vi "加载流程文件.vi"(8 "错误输入（无错误）":errorcluster) -> (0 "错误输出":errorcluster, 3 "流程":T1 {"进样流程"."进样流程-进样"."步骤二："."功能" items=["加标", "进样", "排液", "搅拌", "定量", "延时"]; "进样流程"."进样流程-进样"."步骤一："."功能" items=["加标", "进样", "排液", "搅拌", "定量", "延时"]; "进样流程"."进样流程-进样"."步骤四："."功能" items=["加标", "进样", "排液", "搅拌", "定量", "延时"]; "进样流程"."进样流程-进样"."步骤三："."功能" items=["加标", "进样", "排液", "搅拌", "定量", "延时"]; "进样流程"."进样流程-进样"."步骤六："."功能" items=["加标", "进样", "排液", "搅拌", "定量", "延时"]; "进样流程"."进样流程-进样"."步骤五："."功能" items=["加标", "进样", "排液", "搅拌", "定量", "延时"]; "进样流程"."进样流程-进样"."步骤八："."功能" items=["加标", "进样", "排液", "搅拌", "定量", "延时"]; "进样流程"."进样流程-进样"."步骤七："."功能" items=["加标", "进样", "排液", "搅拌", "定量", "延时"]; "进样流程"."进样流程-进样"."步骤十："."功能" items=["加标", "进样", "排液", "搅拌", "定量", "延时"]; "进样流程"."进样流程-进样"."步骤九："."功能" items=["加标", "进样", "排液", "搅拌", "定量", "延时"]; "进样流程"."进样流程-润洗"."步骤二："."功能" items=["加标", "进样", "排液", "搅拌", "定量", "延时"]; "进样流程"."进样流程-润洗"."步骤一："."功能" items=["加标", "进样", "排液", "搅拌", "定量", "延时"]; "进样流程"."进样流程-润洗"."步骤四："."功能" items=["加标", "进样", "排液", "搅拌", "定量", "延时"]; "进样流程"."进样流程-润洗"."步骤三："."功能" items=["加标", "进样", "排液", "搅拌", "定量", "延时"]; "进样流程"."进样流程-润洗"."步骤六："."功能" items=["加标", "进样", "排液", "搅拌", "定量", "延时"]; "进样流程"."进样流程-润洗"."步骤五："."功能" items=["加标", "进样", "排液", "搅拌", "定量", "延时"]; "进样流程"."进样流程-润洗"."步骤八："."功能" items=["加标", "进样", "排液", "搅拌", "定量", "延时"]; "进样流程"."进样流程-润洗"."步骤七："."功能" items=["加标", "进样", "排液", "搅拌", "定量", "延时"]; "进样流程"."进样流程-润洗"."步骤十："."功能" items=["加标", "进样", "排液", "搅拌", "定量", "延时"]; "进样流程"."进样流程-润洗"."步骤九："."功能" items=["加标", "进样", "排液", "搅拌", "定量", "延时"]; "排液流程"."步骤二："."功能" items=["加标", "进样", "排液", "搅拌", "定量", "延时"]; "排液流程"."步骤一："."功能" items=["加标", "进样", "排液", "搅拌", "定量", "延时"]; "排液流程"."步骤四："."功能" items=["加标", "进样", "排液", "搅拌", "定量", "延时"]; "排液流程"."步骤三："."功能" items=["加标", "进样", "排液", "搅拌", "定量", "延时"]; "排液流程"."步骤六："."功能" items=["加标", "进样", "排液", "搅拌", "定量", "延时"]; "排液流程"."步骤五："."功能" items=["加标", "进样", "排液", "搅拌", "定量", "延时"]; "排液流程"."步骤八："."功能" items=["加标", "进样", "排液", "搅拌", "定量", "延时"]; "排液流程"."步骤七："."功能" items=["加标", "进样", "排液", "搅拌", "定量", "延时"]; "排液流程"."步骤十："."功能" items=["加标", "进样", "排液", "搅拌", "定量", "延时"]; "排液流程"."步骤九："."功能" items=["加标", "进样", "排液", "搅拌", "定量", "延时"]; "加标流程"."加标流程-加标"."步骤二："."功能" items=["加标", "进样", "排液", "搅拌", "定量", "延时"]; "加标流程"."加标流程-加标"."步骤一："."功能" items=["加标", "进样", "排液", "搅拌", "定量", "延时"]; "加标流程"."加标流程-加标"."步骤四："."功能" items=["加标", "进样", "排液", "搅拌", "定量", "延时"]; "加标流程"."加标流程-加标"."步骤三："."功能" items=["加标", "进样", "排液", "搅拌", "定量", "延时"]; "加标流程"."加标流程-加标"."步骤六："."功能" items=["加标", "进样", "排液", "搅拌", "定量", "延时"]; "加标流程"."加标流程-加标"."步骤五："."功能" items=["加标", "进样", "排液", "搅拌", "定量", "延时"]; "加标流程"."加标流程-加标"."步骤八："."功能" items=["加标", "进样", "排液", "搅拌", "定量", "延时"]; "加标流程"."加标流程-加标"."步骤七："."功能" items=["加标", "进样", "排液", "搅拌", "定量", "延时"]; "加标流程"."加标流程-加标"."步骤十："."功能" items=["加标", "进样", "排液", "搅拌", "定量", "延时"]; "加标流程"."加标流程-加标"."步骤九："."功能" items=["加标", "进样", "排液", "搅拌", "定量", "延时"]; "加标流程"."加标流程-定量"."步骤二："."功能" items=["加标", "进样", "排液", "搅拌", "定量", "延时"]; "加标流程"."加标流程-定量"."步骤一："."功能" items=["加标", "进样", "排液", "搅拌", "定量", "延时"]; "加标流程"."加标流程-定量"."步骤四："."功能" items=["加标", "进样", "排液", "搅拌", "定量", "延时"]; "加标流程"."加标流程-定量"."步骤三："."功能" items=["加标", "进样", "排液", "搅拌", "定量", "延时"]; "加标流程"."加标流程-定量"."步骤六："."功能" items=["加标", "进样", "排液", "搅拌", "定量", "延时"]; "加标流程"."加标流程-定量"."步骤五："."功能" items=["加标", "进样", "排液", "搅拌", "定量", "延时"]; "加标流程"."加标流程-定量"."步骤八："."功能" items=["加标", "进样", "排液", "搅拌", "定量", "延时"]; "加标流程"."加标流程-定量"."步骤七："."功能" items=["加标", "进样", "排液", "搅拌", "定量", "延时"]; "加标流程"."加标流程-定量"."步骤十："."功能" items=["加标", "进样", "排液", "搅拌", "定量", "延时"]; "加标流程"."加标流程-定量"."步骤九："."功能" items=["加标", "进样", "排液", "搅拌", "定量", "延时"]; "加标流程"."加标流程-进样"."步骤二："."功能" items=["加标", "进样", "排液", "搅拌", "定量", "延时"]; "加标流程"."加标流程-进样"."步骤一："."功能" items=["加标", "进样", "排液", "搅拌", "定量", "延时"]; "加标流程"."加标流程-进样"."步骤四："."功能" items=["加标", "进样", "排液", "搅拌", "定量", "延时"]; "加标流程"."加标流程-进样"."步骤三："."功能" items=["加标", "进样", "排液", "搅拌", "定量", "延时"]; "加标流程"."加标流程-进样"."步骤六："."功能" items=["加标", "进样", "排液", "搅拌", "定量", "延时"]; "加标流程"."加标流程-进样"."步骤五："."功能" items=["加标", "进样", "排液", "搅拌", "定量", "延时"]; "加标流程"."加标流程-进样"."步骤八："."功能" items=["加标", "进样", "排液", "搅拌", "定量", "延时"]; "加标流程"."加标流程-进样"."步骤七："."功能" items=["加标", "进样", "排液", "搅拌", "定量", "延时"]; "加标流程"."加标流程-进样"."步骤十："."功能" items=["加标", "进样", "排液", "搅拌", "定量", "延时"]; "加标流程"."加标流程-进样"."步骤九："."功能" items=["加标", "进样", "排液", "搅拌", "定量", "延时"]; "加标流程"."加标流程-润洗"."步骤二："."功能" items=["加标", "进样", "排液", "搅拌", "定量", "延时"]; "加标流程"."加标流程-润洗"."步骤一："."功能" items=["加标", "进样", "排液", "搅拌", "定量", "延时"]; "加标流程"."加标流程-润洗"."步骤四："."功能" items=["加标", "进样", "排液", "搅拌", "定量", "延时"]; "加标流程"."加标流程-润洗"."步骤三："."功能" items=["加标", "进样", "排液", "搅拌", "定量", "延时"]; "加标流程"."加标流程-润洗"."步骤六："."功能" items=["加标", "进样", "排液", "搅拌", "定量", "延时"]; "加标流程"."加标流程-润洗"."步骤五："."功能" items=["加标", "进样", "排液", "搅拌", "定量", "延时"]; "加标流程"."加标流程-润洗"."步骤八："."功能" items=["加标", "进样", "排液", "搅拌", "定量", "延时"]; "加标流程"."加标流程-润洗"."步骤七："."功能" items=["加标", "进样", "排液", "搅拌", "定量", "延时"]; "加标流程"."加标流程-润洗"."步骤十："."功能" items=["加标", "进样", "排液", "搅拌", "定量", "延时"]; "加标流程"."加标流程-润洗"."步骤九："."功能" items=["加标", "进样", "排液", "搅拌", "定量", "延时"]; "加标润洗流程"."步骤二："."功能" items=["加标", "进样", "排液", "搅拌", "定量", "延时"]; "加标润洗流程"."步骤一："."功能" items=["加标", "进样", "排液", "搅拌", "定量", "延时"]; "加标润洗流程"."步骤四："."功能" items=["加标", "进样", "排液", "搅拌", "定量", "延时"]; "加标润洗流程"."步骤三："."功能" items=["加标", "进样", "排液", "搅拌", "定量", "延时"]; "加标润洗流程"."步骤六："."功能" items=["加标", "进样", "排液", "搅拌", "定量", "延时"]; "加标润洗流程"."步骤五："."功能" items=["加标", "进样", "排液", "搅拌", "定量", "延时"]; "加标润洗流程"."步骤八："."功能" items=["加标", "进样", "排液", "搅拌", "定量", "延时"]; "加标润洗流程"."步骤七："."功能" items=["加标", "进样", "排液", "搅拌", "定量", "延时"]; "加标润洗流程"."步骤十："."功能" items=["加标", "进样", "排液", "搅拌", "定量", "延时"]; "加标润洗流程"."步骤九："."功能" items=["加标", "进样", "排液", "搅拌", "定量", "延时"]; "水样润洗流程"."步骤二："."功能" items=["加标", "进样", "排液", "搅拌", "定量", "延时"]; "水样润洗流程"."步骤一："."功能" items=["加标", "进样", "排液", "搅拌", "定量", "延时"]; "水样润洗流程"."步骤四："."功能" items=["加标", "进样", "排液", "搅拌", "定量", "延时"]; "水样润洗流程"."步骤三："."功能" items=["加标", "进样", "排液", "搅拌", "定量", "延时"]; "水样润洗流程"."步骤六："."功能" items=["加标", "进样", "排液", "搅拌", "定量", "延时"]; "水样润洗流程"."步骤五："."功能" items=["加标", "进样", "排液", "搅拌", "定量", "延时"]; "水样润洗流程"."步骤八："."功能" items=["加标", "进样", "排液", "搅拌", "定量", "延时"]; "水样润洗流程"."步骤七："."功能" items=["加标", "进样", "排液", "搅拌", "定量", "延时"]; "水样润洗流程"."步骤十："."功能" items=["加标", "进样", "排液", "搅拌", "定量", "延时"]; "水样润洗流程"."步骤九："."功能" items=["加标", "进样", "排液", "搅拌", "定量", "延时"]})   [LabVIEW 2016, in "质控单元V1.lvlib"]
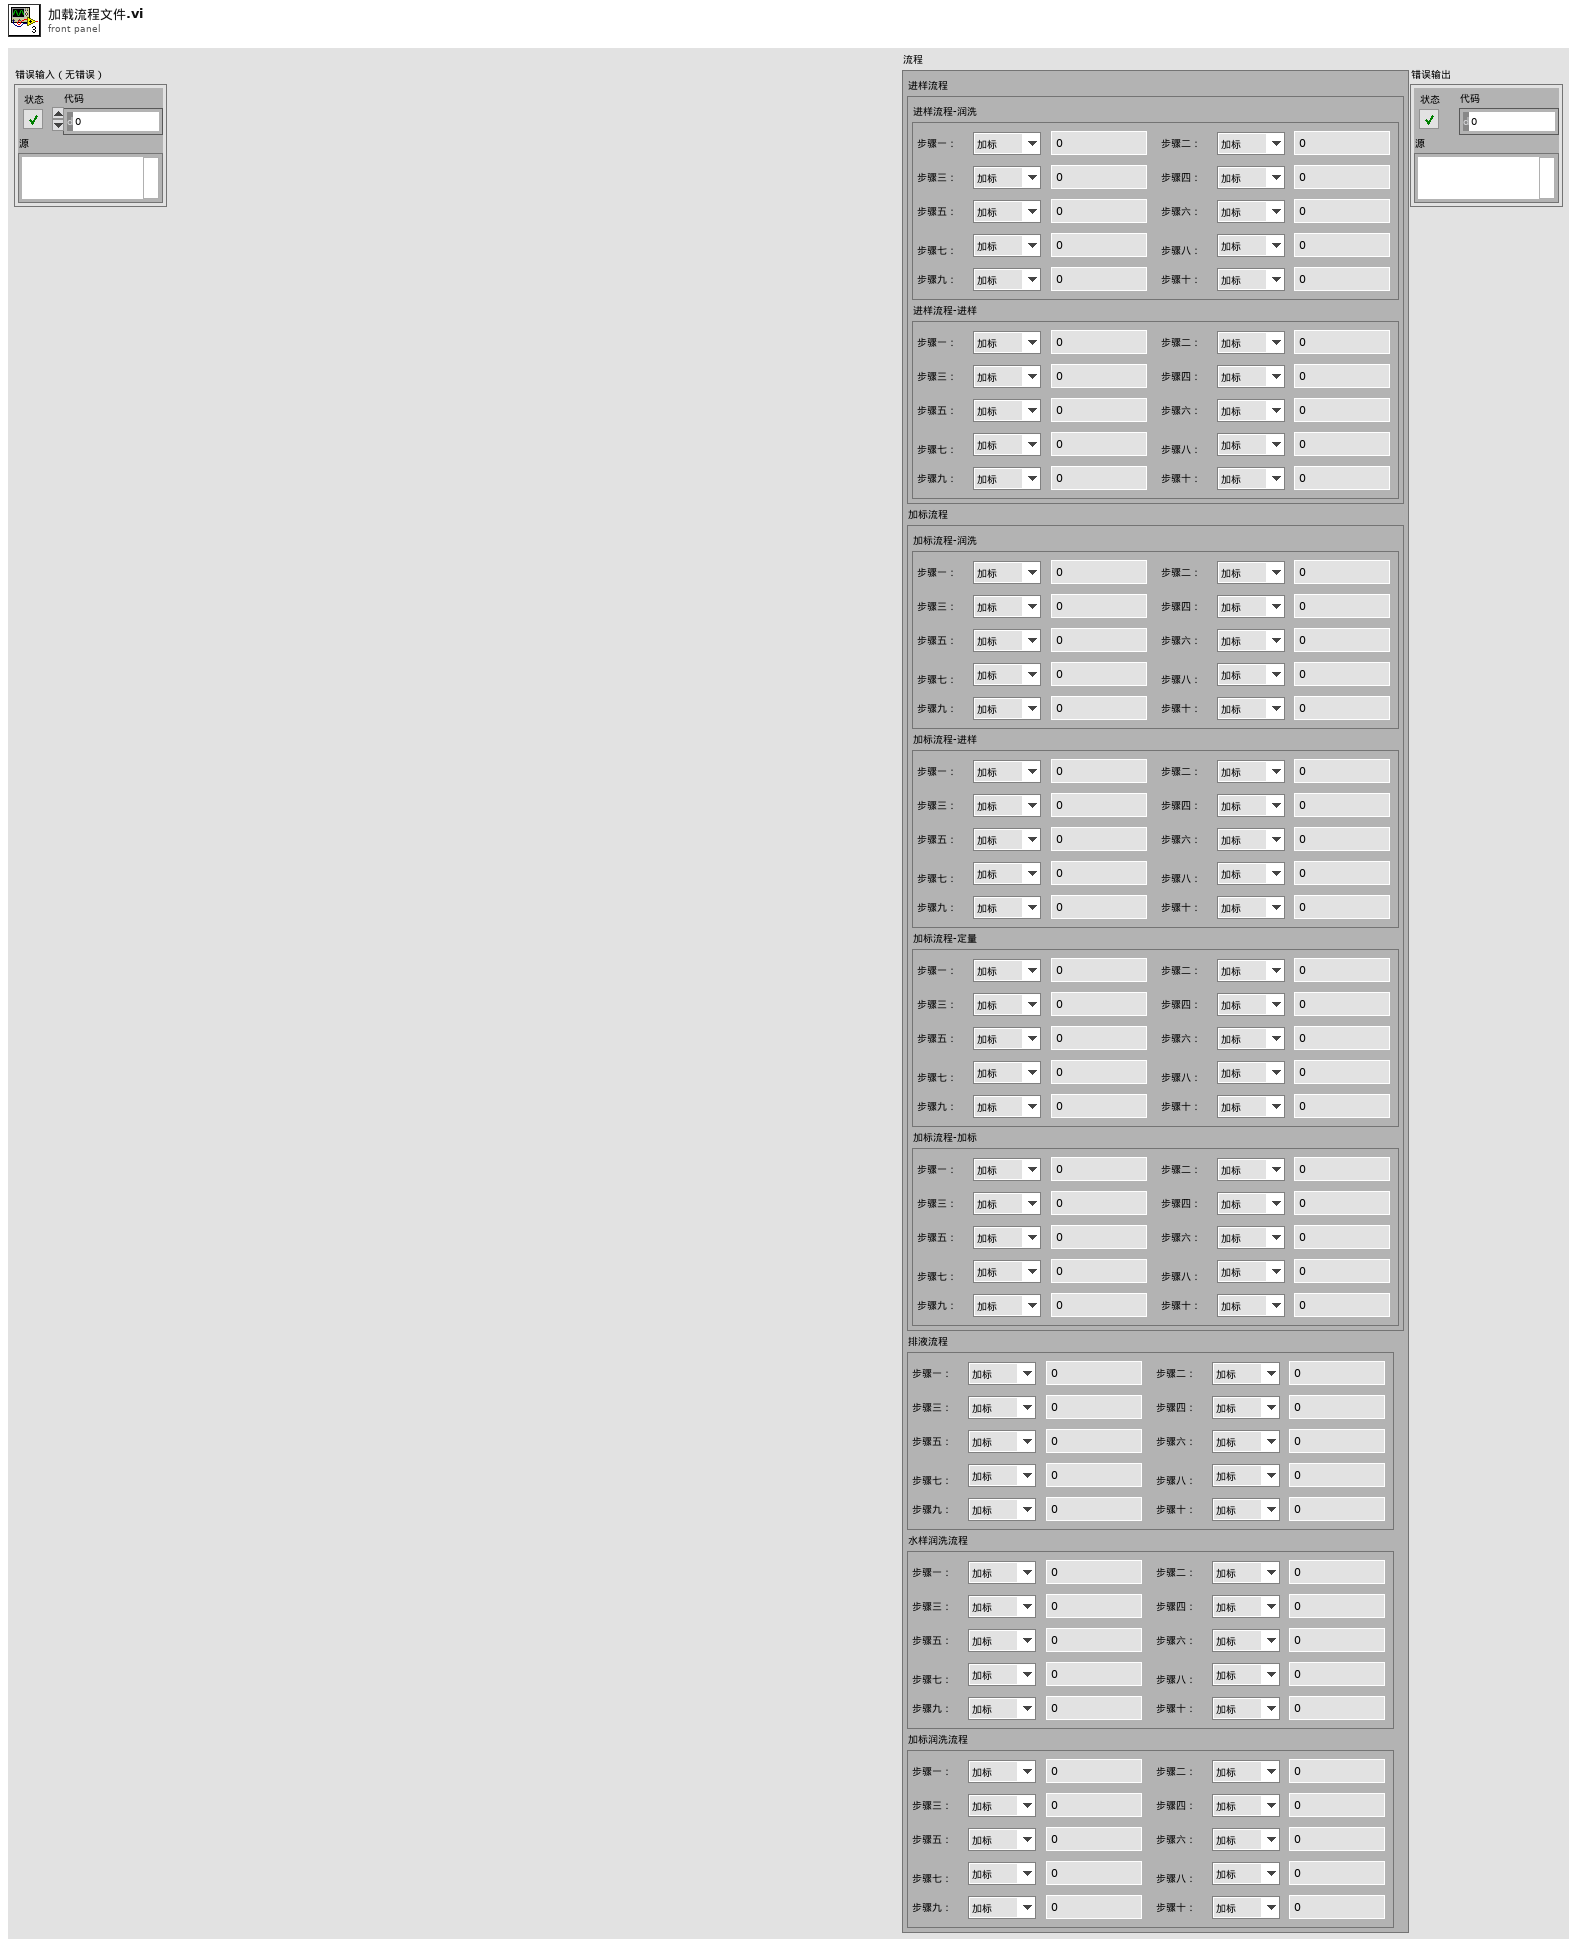
[diagram p1: front panel]
types:
  T1 = cluster{"进样流程":cluster{"进样流程-润洗":cluster{"步骤一：":cluster{"功能":u16, "值":sgl}, "步骤二：":cluster{"功能":u16, "值":sgl}, "步骤三：":cluster{"功能":u16, "值":sgl}, "步骤四：":cluster{"功能":u16, "值":sgl}, "步骤五：":cluster{"功能":u16, "值":sgl}, "步骤六：":cluster{"功能":u16, "值":sgl}, "步骤七：":cluster{"功能":u16, "值":sgl}, "步骤八：":cluster{"功能":u16, "值":sgl}, "步骤九：":cluster{"功能":u16, "值":sgl}, "步骤十：":cluster{"功能":u16, "值":sgl}}, "进样流程-进样":cluster{"步骤一：":cluster{"功能":u16, "值":sgl}, "步骤二：":cluster{"功能":u16, "值":sgl}, "步骤三：":cluster{"功能":u16, "值":sgl}, "步骤四：":cluster{"功能":u16, "值":sgl}, "步骤五：":cluster{"功能":u16, "值":sgl}, "步骤六：":cluster{"功能":u16, "值":sgl}, "步骤七：":cluster{"功能":u16, "值":sgl}, "步骤八：":cluster{"功能":u16, "值":sgl}, "步骤九：":cluster{"功能":u16, "值":sgl}, "步骤十：":cluster{"功能":u16, "值":sgl}}}, "加标流程":cluster{"加标流程-润洗":cluster{"步骤一：":cluster{"功能":u16, "值":sgl}, "步骤二：":cluster{"功能":u16, "值":sgl}, "步骤三：":cluster{"功能":u16, "值":sgl}, "步骤四：":cluster{"功能":u16, "值":sgl}, "步骤五：":cluster{"功能":u16, "值":sgl}, "步骤六：":cluster{"功能":u16, "值":sgl}, "步骤七：":cluster{"功能":u16, "值":sgl}, "步骤八：":cluster{"功能":u16, "值":sgl}, "步骤九：":cluster{"功能":u16, "值":sgl}, "步骤十：":cluster{"功能":u16, "值":sgl}}, "加标流程-进样":cluster{"步骤一：":cluster{"功能":u16, "值":sgl}, "步骤二：":cluster{"功能":u16, "值":sgl}, "步骤三：":cluster{"功能":u16, "值":sgl}, "步骤四：":cluster{"功能":u16, "值":sgl}, "步骤五：":cluster{"功能":u16, "值":sgl}, "步骤六：":cluster{"功能":u16, "值":sgl}, "步骤七：":cluster{"功能":u16, "值":sgl}, "步骤八：":cluster{"功能":u16, "值":sgl}, "步骤九：":cluster{"功能":u16, "值":sgl}, "步骤十：":cluster{"功能":u16, "值":sgl}}, "加标流程-定量":cluster{"步骤一：":cluster{"功能":u16, "值":sgl}, "步骤二：":cluster{"功能":u16, "值":sgl}, "步骤三：":cluster{"功能":u16, "值":sgl}, "步骤四：":cluster{"功能":u16, "值":sgl}, "步骤五：":cluster{"功能":u16, "值":sgl}, "步骤六：":cluster{"功能":u16, "值":sgl}, "步骤七：":cluster{"功能":u16, "值":sgl}, "步骤八：":cluster{"功能":u16, "值":sgl}, "步骤九：":cluster{"功能":u16, "值":sgl}, "步骤十：":cluster{"功能":u16, "值":sgl}}, "加标流程-加标":cluster{"步骤一：":cluster{"功能":u16, "值":sgl}, "步骤二：":cluster{"功能":u16, "值":sgl}, "步骤三：":cluster{"功能":u16, "值":sgl}, "步骤四：":cluster{"功能":u16, "值":sgl}, "步骤五：":cluster{"功能":u16, "值":sgl}, "步骤六：":cluster{"功能":u16, "值":sgl}, "步骤七：":cluster{"功能":u16, "值":sgl}, "步骤八：":cluster{"功能":u16, "值":sgl}, "步骤九：":cluster{"功能":u16, "值":sgl}, "步骤十：":cluster{"功能":u16, "值":sgl}}}, "排液流程":cluster{"步骤一：":cluster{"功能":u16, "值":sgl}, "步骤二：":cluster{"功能":u16, "值":sgl}, "步骤三：":cluster{"功能":u16, "值":sgl}, "步骤四：":cluster{"功能":u16, "值":sgl}, "步骤五：":cluster{"功能":u16, "值":sgl}, "步骤六：":cluster{"功能":u16, "值":sgl}, "步骤七：":cluster{"功能":u16, "值":sgl}, "步骤八：":cluster{"功能":u16, "值":sgl}, "步骤九：":cluster{"功能":u16, "值":sgl}, "步骤十：":cluster{"功能":u16, "值":sgl}}, "水样润洗流程":cluster{"步骤一：":cluster{"功能":u16, "值":sgl}, "步骤二：":cluster{"功能":u16, "值":sgl}, "步骤三：":cluster{"功能":u16, "值":sgl}, "步骤四：":cluster{"功能":u16, "值":sgl}, "步骤五：":cluster{"功能":u16, "值":sgl}, "步骤六：":cluster{"功能":u16, "值":sgl}, "步骤七：":cluster{"功能":u16, "值":sgl}, "步骤八：":cluster{"功能":u16, "值":sgl}, "步骤九：":cluster{"功能":u16, "值":sgl}, "步骤十：":cluster{"功能":u16, "值":sgl}}, "加标润洗流程":cluster{"步骤一：":cluster{"功能":u16, "值":sgl}, "步骤二：":cluster{"功能":u16, "值":sgl}, "步骤三：":cluster{"功能":u16, "值":sgl}, "步骤四：":cluster{"功能":u16, "值":sgl}, "步骤五：":cluster{"功能":u16, "值":sgl}, "步骤六：":cluster{"功能":u16, "值":sgl}, "步骤七：":cluster{"功能":u16, "值":sgl}, "步骤八：":cluster{"功能":u16, "值":sgl}, "步骤九：":cluster{"功能":u16, "值":sgl}, "步骤十：":cluster{"功能":u16, "值":sgl}}}
  T2 = cluster{"flow1":cluster{"Type":u16, "Value":sgl}[], "flow2":cluster{"Type":u16, "Value":sgl}[], "flow3":cluster{"Type":u16, "Value":sgl}[], "flow4":cluster{"Type":u16, "Value":sgl}[], "flow5":cluster{"Type":u16, "Value":sgl}[]}
  T3 = cluster{"[0]":cluster{"Type":u16, "Value":sgl}, "[1]":cluster{"Type":u16, "Value":sgl}, "[2]":cluster{"Type":u16, "Value":sgl}, "[3]":cluster{"Type":u16, "Value":sgl}, "[4]":cluster{"Type":u16, "Value":sgl}, "[5]":cluster{"Type":u16, "Value":sgl}, "[6]":cluster{"Type":u16, "Value":sgl}, "[7]":cluster{"Type":u16, "Value":sgl}, "[8]":cluster{"Type":u16, "Value":sgl}, "[9]":cluster{"Type":u16, "Value":sgl}}
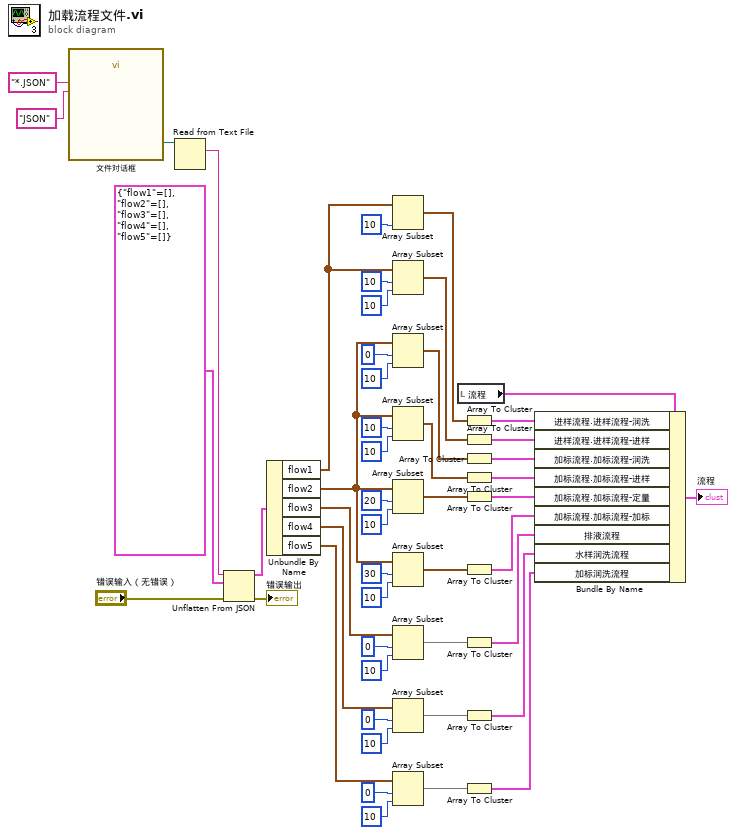
[diagram p0: block diagram]
diagram:
  n1 = call "文件对话框"("pattern (all files)"="*.JSON", "pattern label"="JSON") -> ("selected path"=w49:path)  [unwired: 10 in, 3 out]
  n2 = Read from Text File(file (use dialog)=w49) -> (text=w48:string)  [unwired: 3 in, 3 out]
  n3 = Unflatten From JSON(JSON string=w48, type and defaults=T2 {"flow1"=[], "flow2"=[], "flow3"=[], "flow4"=[], "flow5"=[]}, error in (no error)="错误输入（无错误）") -> (value=w45:T2, error out=→"错误输出":errorcluster)  [unwired: 4 in]
  n4 = Unbundle By Name(w45) -> ("flow1"=w38:cluster{"Type":u16, "Value":sgl}[], "flow2"=w21:cluster{"Type":u16, "Value":sgl}[], "flow3"=w14:cluster{"Type":u16, "Value":sgl}[], "flow4"=w9:cluster{"Type":u16, "Value":sgl}[], "flow5"=w4:cluster{"Type":u16, "Value":sgl}[])
  n5 = Array Subset(array=w38, length=10 ("长度")) -> (w41:cluster{"Type":u16, "Value":sgl}[])  [unwired: 1 in]
  n6 = Array Subset(array=w38, index=10 ("索引"), length=10 ("长度")) -> (w37:cluster{"Type":u16, "Value":sgl}[])
  n7 = Array Subset(array=w21, index=0 ("索引"), length=10 ("长度")) -> (w32:cluster{"Type":u16, "Value":sgl}[])
  n8 = Array Subset(array=w21, index=10 ("索引"), length=10 ("长度")) -> (w30:cluster{"Type":u16, "Value":sgl}[])
  n9 = Array Subset(array=w21, index=20 ("索引"), length=10 ("长度")) -> (w25:cluster{"Type":u16, "Value":sgl}[])
  n10 = Array Subset(array=w21, index=30 ("索引"), length=10 ("长度")) -> (w24:cluster{"Type":u16, "Value":sgl}[])
  n11 = Array Subset(array=w14, index=0 ("索引"), length=10 ("长度")) -> (w15:cluster{"Type":u16, "Value":sgl}[])
  n12 = Array Subset(array=w9, index=0 ("索引"), length=10 ("长度")) -> (w12:cluster{"Type":u16, "Value":sgl}[])
  n13 = Array Subset(array=w4, index=0 ("索引"), length=10 ("长度")) -> (w5:cluster{"Type":u16, "Value":sgl}[])
  n14 = local read "流程"() -> (w44:T1)
  n15 = Array To Cluster(array=w41) -> (cluster=w40:T3)
  n16 = Array To Cluster(array=w37) -> (cluster=w36:T3)
  n17 = Array To Cluster(array=w32) -> (cluster=w31:T3)
  n18 = Array To Cluster(array=w30) -> (cluster=w20:T3)
  n19 = Array To Cluster(array=w25) -> (cluster=w19:T3)
  n20 = Array To Cluster(array=w24) -> (cluster=w18:T3)
  n21 = Array To Cluster(array=w15) -> (cluster=w13:T3)
  n22 = Array To Cluster(array=w12) -> (cluster=w8:T3)
  n23 = Array To Cluster(array=w5) -> (cluster=w3:T3)
  n24 = Bundle By Name(cluster=w44, "进样流程.进样流程-润洗"=w40, "进样流程.进样流程-进样"=w36, "加标流程.加标流程-润洗"=w31, "加标流程.加标流程-进样"=w20, "加标流程.加标流程-定量"=w19, "加标流程.加标流程-加标"=w18, "排液流程"=w13, "水样润洗流程"=w8, "加标润洗流程"=w3) -> (→"流程":T1)
